vi "GetAccelerometerData.vi"(0 "LINX Resource":T2, 1 "input Mag":T1, 3 "I2C Channel (0)":u8, 5 "Chip":enum16{"LSM6DS1", "LSM6DS3", "ADXL345"}(ring), 9 "alpha":dbl=0.5 format="%#_13g", 11 "Error In":errorcluster, 12 "input Gs":T1) -> (4 "LINX Resource":T2, 6 "G-Filtered":T1, 8 "Mag-Filtered":T1, 10 "Roll Pitch Yaw":T1, 15 "Error Out":errorcluster)   [LabVIEW 2014]
uses:
  <vilib>/LabVIEW Hacker/LINX/Private/Type Defs/LINX Ref.ctl
  <vilib>/LabVIEW Hacker/LINX/Private/Type Defs/Platform.ctl
  <vilib>/LabVIEW Hacker/LINX/Private/Type Defs/Interface.ctl
  <vilib>/LabVIEW Hacker/LINX/Private/Device/Type Defs/LINX Device Config.ctl
  <vilib>/LabVIEW Hacker/LINX/Private/Device/Type Defs/TCP Config.ctl
  <vilib>/LabVIEW Hacker/LINX/Private/Type Defs/Device Family.ctl
  <vilib>/LabVIEW Hacker/LINX/LVH-LINX.lvlib
  <vilib>/LabVIEW Hacker/LVH-Toolbox/Common/LVH-Common.lvlib
  <vilib>/LabVIEW Hacker/LINX/Private/Device/Device.lvlib
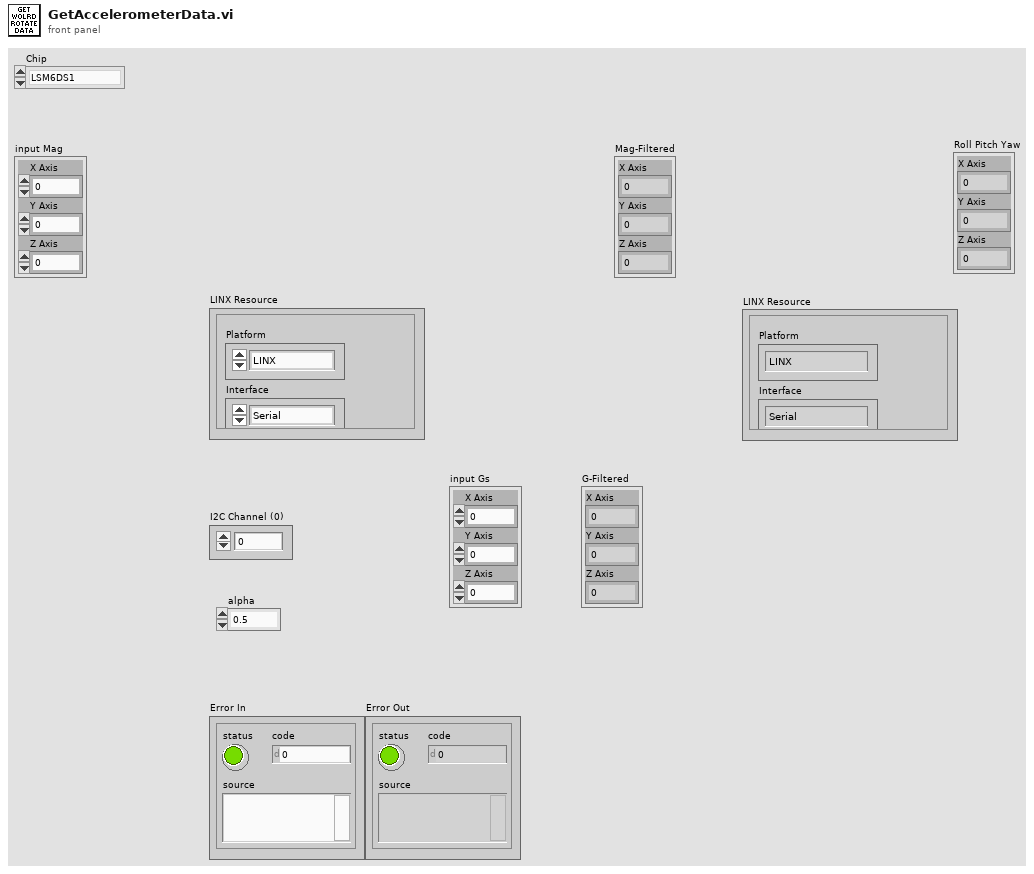
[diagram p1: front panel]
types:
  T1 = cluster{"X Axis":dbl, "Y Axis":dbl, "Z Axis":dbl}
  T2 = typedef "LVH-LINX.lvlib/LINX Ref.ctl" = cluster{"Platform":T3, "Interface":T4, "LINX Device Config":T5}
  T3 = typedef "LVH-LINX.lvlib/Platform.ctl" = enum16{"LINX", "myRIO"}
  T4 = typedef "LVH-LINX.lvlib/Interface.ctl" = enum16{"Serial", "TCP"}
  T5 = typedef "LVH-LINX.lvlib/Device.lvlib/LINX Device Config.ctl" = cluster{"Interface":T4, "COM Port":refnum<visa-resource-name>, "TCP Configuration":T6, "Device Family":T7, "Device ID":u8, "Device Name":string, "TCP Ref":refnum<k5>}
  T6 = typedef "LVH-LINX.lvlib/Device.lvlib/TCP Config.ctl" = cluster{"IP Address":string, "Port":u16}
  T7 = typedef "LVH-LINX.lvlib/Device Family.ctl" = enum8{"National Instruments", "Digilent", "Arduino"}
  T8 = cluster{"Decimal I16":i16, "Decimal I16":i16, "Decimal I16":i16}
  T9 = cluster{"Decimal I16":dbl, "Decimal I16":dbl, "Decimal I16":dbl}
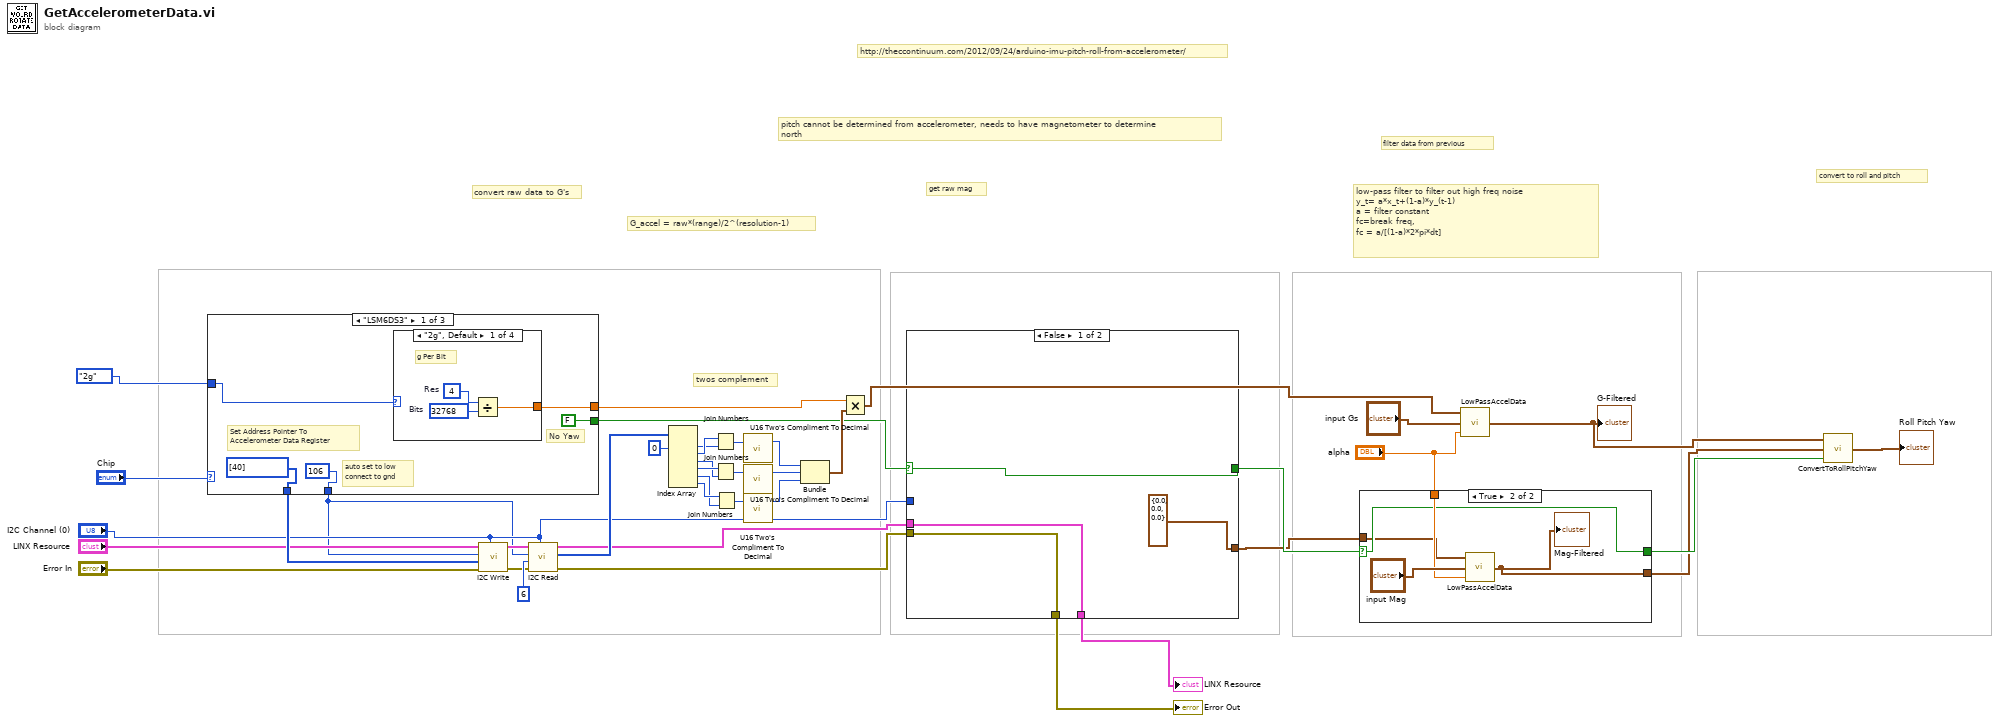
[diagram p0: block diagram]
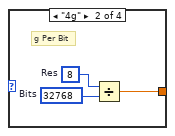
[diagram p2: hidden frame]
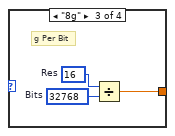
[diagram p3: hidden frame]
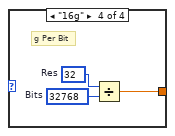
[diagram p4: hidden frame]
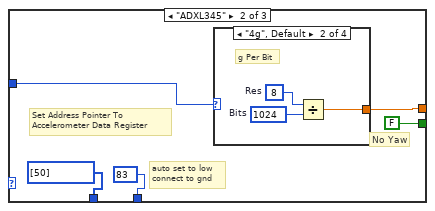
[diagram p5: hidden frame]
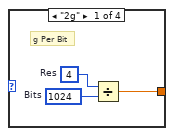
[diagram p6: hidden frame]
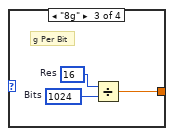
[diagram p7: hidden frame]
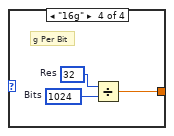
[diagram p8: hidden frame]
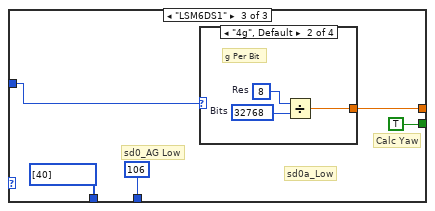
[diagram p9: hidden frame]
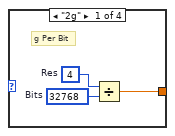
[diagram p10: hidden frame]
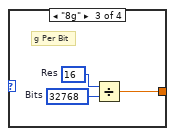
[diagram p11: hidden frame]
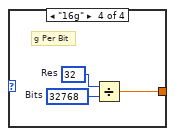
[diagram p12: hidden frame]
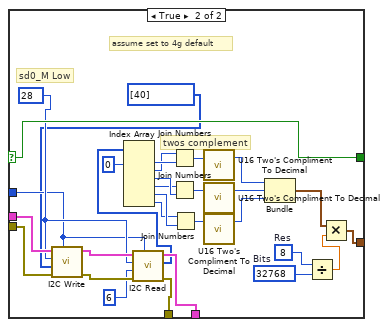
[diagram p13: hidden frame]
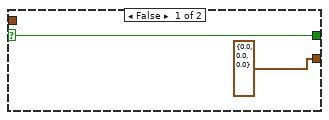
[diagram p14: hidden frame]
diagram:
  # "twos complement"
  # "G_accel = raw*(range)/2^(resolution-1)"
  # "get raw mag"
  # "convert to roll and pitch"
  # "filter data from previous"
  # "convert raw data to G's"
  # "http://theccontinuum.com/2012/09/24/arduino-imu-pitch-roll-from-accelerometer/"
  # "low-pass filter to filter out high freq noise\ny_t= a*x_t+(1-a)*y_(t-1)\na = filter constant\nfc=break freq,\nfc = a/[(1-a)*2*pi*dt]"
  # "pitch cannot be determined from accelerometer, needs to have magnetometer to determine north"
  n1 = case shown="\"LSM6DS3\"" "Chip" {
    tunnel: [u8 106 ("I2C Slave Address (0)") u8 83 ("I2C Slave Address (0)") u8 106 ("I2C Slave Address (0)")] -> w1
    tunnel: [u8[] [40] ("Data") u8[] [50] ("Data") u8[] [40] ("Data")] -> w15
    tunnel: [FALSE FALSE TRUE] -> w12
    tunnel: [w42 w59 w76] -> w10
    tunnel: enum16{"2g", "4g", "8g", "16g"}."2g" ("Resolution") -> [w41 w58 w75]
    frame "LSM6DS3" {
      # "No Yaw"
      # "auto set to low\nconnect to gnd"
      # "Set Address Pointer To \nAccelerometer Data Register"
      n2 = case shown="\"2g\", Default" w41 {
        tunnel: [w46 w49 w52 w55] -> w42
        frame "2g", Default {
          w47 = 4  # Res
          w48 = 32768  # Bits
          # "g Per Bit"
          n3 = Divide(x=w47, y=w48) -> (x/y=w46:dbl)
        }
        frame "4g" {
          w50 = 8  # Res
          w51 = 32768  # Bits
          # "g Per Bit"
          n4 = Divide(x=w50, y=w51) -> (x/y=w49:dbl)
        }
        frame "8g" {
          w53 = 16  # Res
          w54 = 32768  # Bits
          # "g Per Bit"
          n5 = Divide(x=w53, y=w54) -> (x/y=w52:dbl)
        }
        frame "16g" {
          w56 = 32  # Res
          w57 = 32768  # Bits
          # "g Per Bit"
          n6 = Divide(x=w56, y=w57) -> (x/y=w55:dbl)
        }
      }
    }
    frame "ADXL345" {
      # "No Yaw"
      # "auto set to low\nconnect to gnd"
      # "Set Address Pointer To \nAccelerometer Data Register"
      n7 = case shown="\"4g\", Default" w58 {
        tunnel: [w63 w66 w69 w72] -> w59
        frame "2g" {
          w64 = 4  # Res
          w65 = 1024  # Bits
          # "g Per Bit"
          n8 = Divide(x=w64, y=w65) -> (x/y=w63:dbl)
        }
        frame "4g", Default {
          w67 = 8  # Res
          w68 = 1024  # Bits
          # "g Per Bit"
          n9 = Divide(x=w67, y=w68) -> (x/y=w66:dbl)
        }
        frame "8g" {
          w70 = 16  # Res
          w71 = 1024  # Bits
          # "g Per Bit"
          n10 = Divide(x=w70, y=w71) -> (x/y=w69:dbl)
        }
        frame "16g" {
          w73 = 32  # Res
          w74 = 1024  # Bits
          # "g Per Bit"
          n11 = Divide(x=w73, y=w74) -> (x/y=w72:dbl)
        }
      }
    }
    frame "LSM6DS1" {
      # "sd0a_Low"
      # "sd0_AG Low"
      # "Calc Yaw"
      n12 = case shown="\"4g\", Default" w75 {
        tunnel: [w80 w83 w86 w89] -> w76
        frame "2g" {
          w81 = 4  # Res
          w82 = 32768  # Bits
          # "g Per Bit"
          n13 = Divide(x=w81, y=w82) -> (x/y=w80:dbl)
        }
        frame "4g", Default {
          w84 = 8  # Res
          w85 = 32768  # Bits
          # "g Per Bit"
          n14 = Divide(x=w84, y=w85) -> (x/y=w83:dbl)
        }
        frame "8g" {
          w87 = 16  # Res
          w88 = 32768  # Bits
          # "g Per Bit"
          n15 = Divide(x=w87, y=w88) -> (x/y=w86:dbl)
        }
        frame "16g" {
          w90 = 32  # Res
          w91 = 32768  # Bits
          # "g Per Bit"
          n16 = Divide(x=w90, y=w91) -> (x/y=w89:dbl)
        }
      }
    }
  }
  n17 = call <vilib>:"I2C Write.vi"("I2C Channel"="I2C Channel (0)", "Error In"="Error In", "Data"=w15, "I2C Slave Address (0)"=w1, "LINX Resource"="LINX Resource") -> ("Error Out"=w16:errorcluster, "LINX Resource"=w17:T2)  [unwired: 5 in]
  n18 = call <vilib>:"I2C Read.vi"("I2C Channel"="I2C Channel (0)", "Error In"=w16, "Bytes To Read"=u8 6, "I2C Slave Address (0)"=w1, "LINX Resource"=w17) -> ("Error Out"=w7:errorcluster, "Data"=w20:u8[], "LINX Resource"=w5:T2)  [unwired: 4 in]
  n19 = Index Array(array=w20, index #1=0 ("index")) -> (element #1=w22:u8, element #2=w23:u8, element #3=w24:u8, element #4=w25:u8, element #5=w26:u8, element #6=w27:u8)  [unwired: 5 in]
  n20 = Join Numbers(hi=w23, lo=w22) -> ((hi.lo)=w28:u16)
  n21 = Join Numbers(hi=w25, lo=w24) -> ((hi.lo)=w29:u16)
  n22 = Join Numbers(hi=w27, lo=w26) -> ((hi.lo)=w30:u16)
  n23 = call <vilib>:"U16 Two's Compliment To Decimal.vi"("Two's Compliment U16"=w28) -> ("Decimal I16"=w31:i16)  [unwired: 2 in]
  n24 = call <vilib>:"U16 Two's Compliment To Decimal.vi"("Two's Compliment U16"=w29) -> ("Decimal I16"=w32:i16)  [unwired: 2 in]
  n25 = call <vilib>:"U16 Two's Compliment To Decimal.vi"("Two's Compliment U16"=w30) -> ("Decimal I16"=w33:i16)  [unwired: 2 in]
  n26 = Bundle("Decimal I16"=w31, "Decimal I16"=w32, "Decimal I16"=w33) -> (w18:T8)  [unwired: 1 in]
  n27 = Multiply(x=w10, y=w18) -> (x*y=w3:T9)
  n28 = case shown="False" w12 {
    selector: w12 -> [w95 w125]
    tunnel: [w95 w125] -> w38
    tunnel: "I2C Channel (0)" -> [_ w98]
    tunnel: w7 -> [w93 w124]
    tunnel: [w93 w116] -> w6
    tunnel: [w94 w118] -> w4
    tunnel: w5 -> [w94 w123]
    tunnel: [T1 {"X Axis"=0.0, "Y Axis"=0.0, "Z Axis"=0.0} ("Mag-Filtered 2") w97] -> w2
    frame False {
    }
    frame True {
      w99 = u8 28 ("I2C Slave Address (0)")
      w122 = 8  # Res
      w121 = 32768  # Bits
      # "twos complement"
      # "assume set to 4g default"
      # "sd0_M Low"
      n29 = call <vilib>:"I2C Write.vi"("I2C Channel"=w98, "Error In"=w124, "Data"=u8[] [40], "I2C Slave Address (0)"=w99, "LINX Resource"=w123) -> ("Error Out"=w117:errorcluster, "LINX Resource"=w119:T2)  [unwired: 5 in]
      n30 = call <vilib>:"I2C Read.vi"("I2C Channel"=w98, "Error In"=w117, "Bytes To Read"=u8 6, "I2C Slave Address (0)"=w99, "LINX Resource"=w119) -> ("Error Out"=w116:errorcluster, "Data"=w101:u8[], "LINX Resource"=w118:T2)  [unwired: 4 in]
      n31 = Index Array(array=w101, index #1=0 ("index")) -> (element #1=w114:u8, element #2=w113:u8, element #3=w112:u8, element #4=w111:u8, element #5=w110:u8, element #6=w109:u8)  [unwired: 5 in]
      n32 = Join Numbers(hi=w113, lo=w114) -> ((hi.lo)=w108:u16)
      n33 = Join Numbers(hi=w111, lo=w112) -> ((hi.lo)=w107:u16)
      n34 = Join Numbers(hi=w109, lo=w110) -> ((hi.lo)=w106:u16)
      n35 = call <vilib>:"U16 Two's Compliment To Decimal.vi"("Two's Compliment U16"=w108) -> ("Decimal I16"=w105:i16)  [unwired: 2 in]
      n36 = call <vilib>:"U16 Two's Compliment To Decimal.vi"("Two's Compliment U16"=w107) -> ("Decimal I16"=w104:i16)  [unwired: 2 in]
      n37 = call <vilib>:"U16 Two's Compliment To Decimal.vi"("Two's Compliment U16"=w106) -> ("Decimal I16"=w103:i16)  [unwired: 2 in]
      n38 = Bundle("Decimal I16"=w105, "Decimal I16"=w104, "Decimal I16"=w103) -> (w102:T8)  [unwired: 1 in]
      n39 = Divide(x=w122, y=w121) -> (x/y=w120:dbl)
      n40 = Multiply(x=w102, y=w120) -> (x*y=w97:T9)
    }
  }
  "LINX Resource" <- w4
  "Error Out" <- w6
  n41 = case shown="True" w38 {
    selector: w38 -> [w127 w130]
    tunnel: "alpha" -> [_ w131]
    tunnel: [w127 w130] -> w36
    tunnel: [T1 {"X Axis"=0.0, "Y Axis"=0.0, "Z Axis"=0.0} ("Mag-Filtered 2") w129] -> w35
    tunnel: w2 -> [_ w128]
    frame False {
    }
    frame True {
      n42 = call "LowPassAccelData.vi"("alpha"=w131, "Prev Gs"="input Mag", "Input Gs"=w128) -> ("G-Filtered"=w129:T1)
      "Mag-Filtered" <- w129
    }
  }
  n43 = call "LowPassAccelData.vi"("alpha"="alpha", "Prev Gs"="input Gs", "Input Gs"=w3) -> ("G-Filtered"=w37:T1)
  "G-Filtered" <- w37
  n44 = call "ConvertToRollPitchYaw.vi"("Yaw"=w36, "Input-Mag"=w35, "Input-Gs"=w37) -> ("Roll Pitch Yaw"=→"Roll Pitch Yaw":T1)
